vi "Main.vi"(0 "Operations":string(combo), 1 "Delete":bool, 2 "Save":bool, 3 "Load":bool, 5 "Add":bool, 7 "Tree":string(tree), 11 "Error In":errorcluster) -> (15 "Error Out":errorcluster)   [LabVIEW 2023]
doc: "The VI adds the selected the operation into the tree and loads the instances which performs the arithmetic operations and it can save or load the class data into the XML files"
uses:
  Typedef/Queue Operation.ctl
  Typedef/Calculator Data.ctl
  Typedef/Class Data.ctl
  Classes/Arithemtic Operation/Arithemetic Operation.lvclass
  Typedef/DVR Ref.ctl
  Typedef/User Event Operations.ctl
  <vilib>/Utility/xml.llb/Write to XML File(string).vi
  <vilib>/Utility/xml.llb/Read From XML File(array).vi
panel:
  # "Instructions:\n1. Run the VI.\n2. Select the operation to be done from the Operations.\n3. Click Add to create a instance and is added in the tree.\n4. Select the instance name in the tree to load the instance.\n5. Specify the input values in the instance and observe the output\n6. On clicking the Delete button the selected instance will be deleted. \n7. Click Save to save the values all instances in an XML file.\n8. Click Load to load the values of all instances from an XML file.\n9. Click panel close to stop the VI from running."
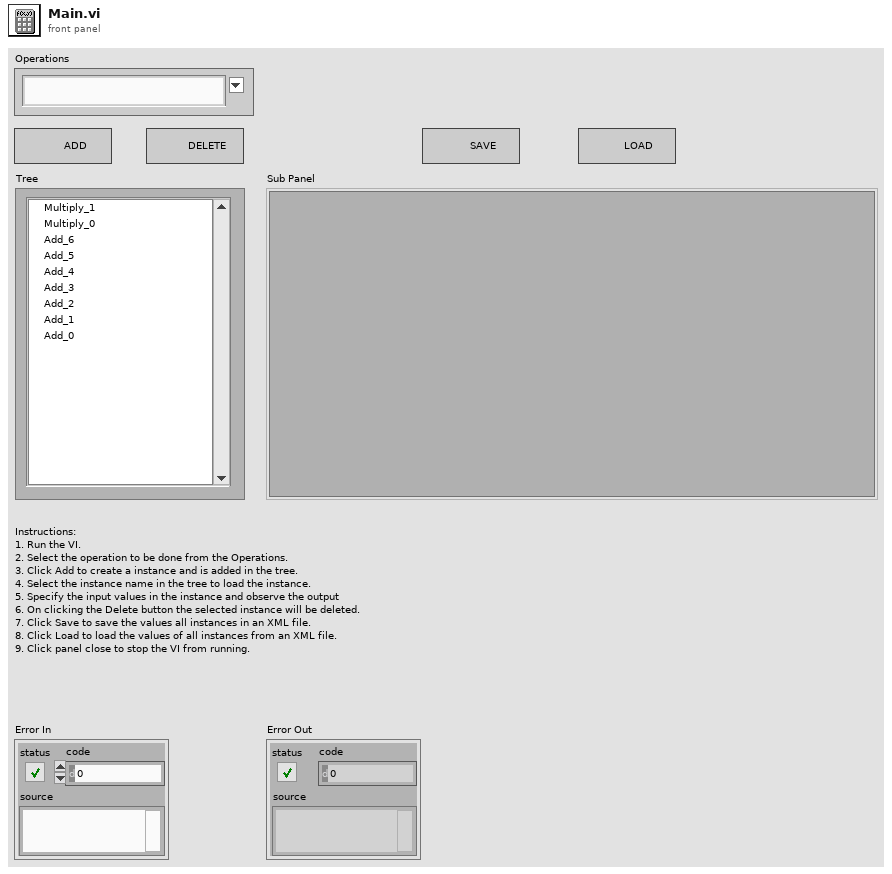
[diagram p1: front panel]
types:
  T1 = typedef "User Event Operations.ctl" = enum16{"Obtain", "Generate", "Release"}
  T2 = typedef "Calculator Data.ctl" = cluster{"Selected Item":string, "Selected Tag":string, "XML Path":path, "Instance Data Array":T3[], "Class Name":string, "Close":refnum<data-value>, "DVR Ref Array":T4[]}
  T3 = typedef "Class Data.ctl" = cluster{"Class Data":refnum<class "Arithemetic Operation.lvclass">, "Name":string}
  T4 = typedef "DVR Ref.ctl" = cluster{"Class Name":string, "DVR":refnum<data-value>}
  T5 = typedef "Queue Operation.ctl" = enum16{"Create & Enqueue N", "Enqueue N", "Dequeue", "Enstack N", "Flush", "Release"}
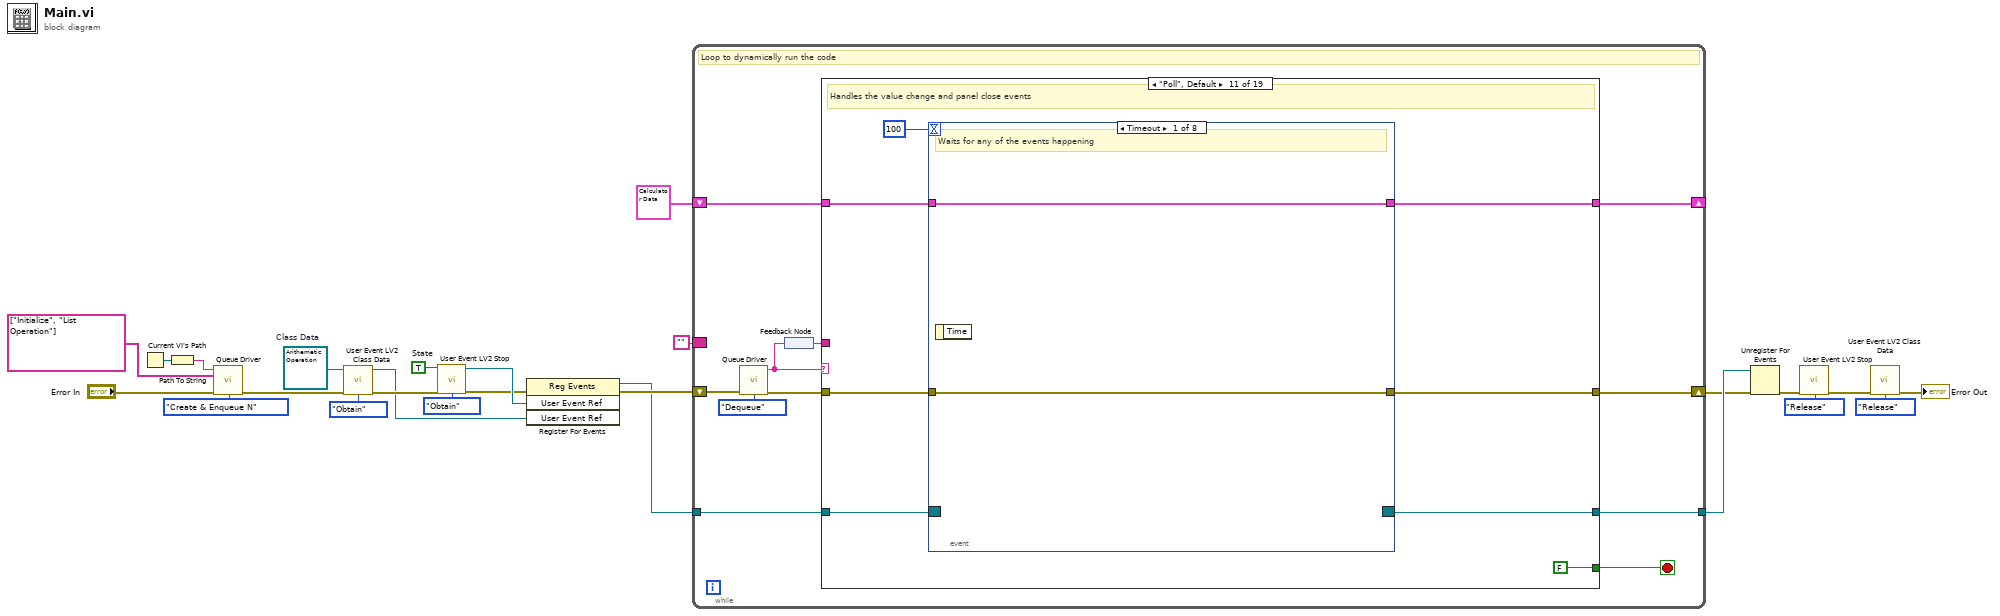
[diagram p0: block diagram]
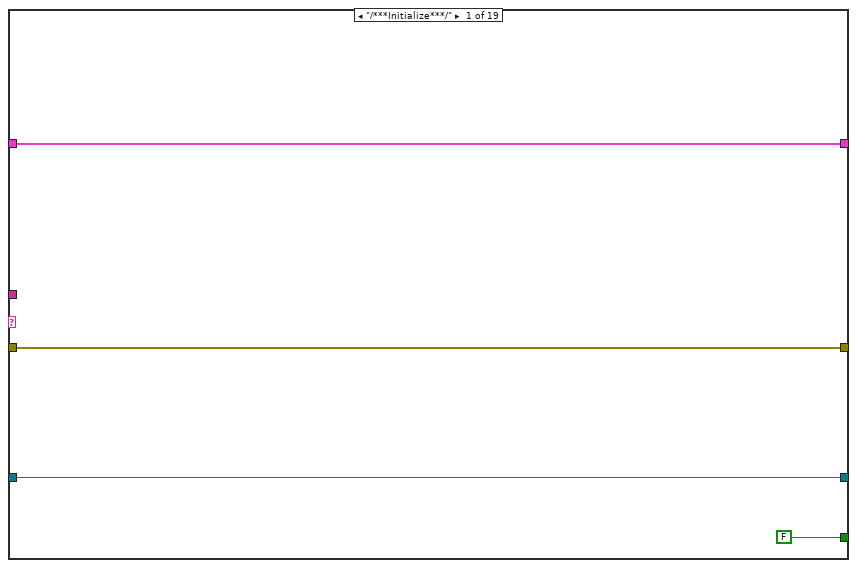
[diagram p2: hidden frame]
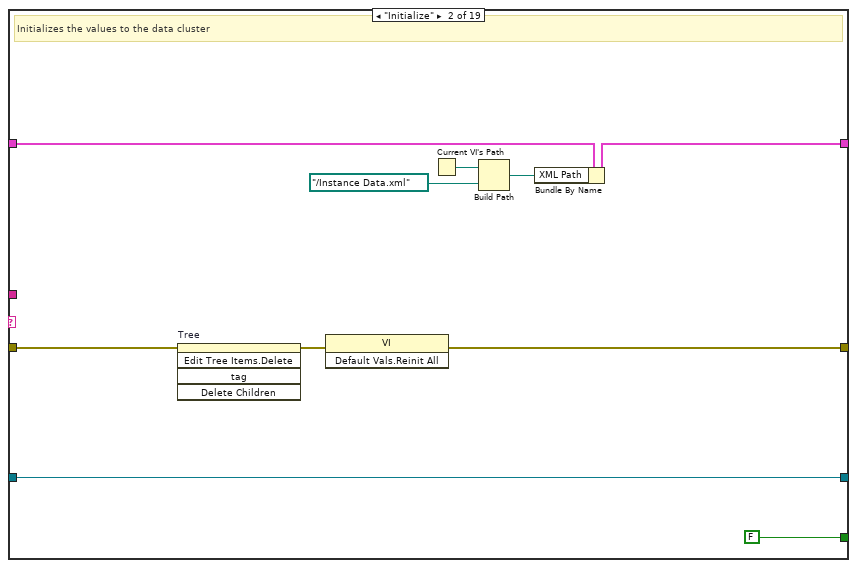
[diagram p3: hidden frame]
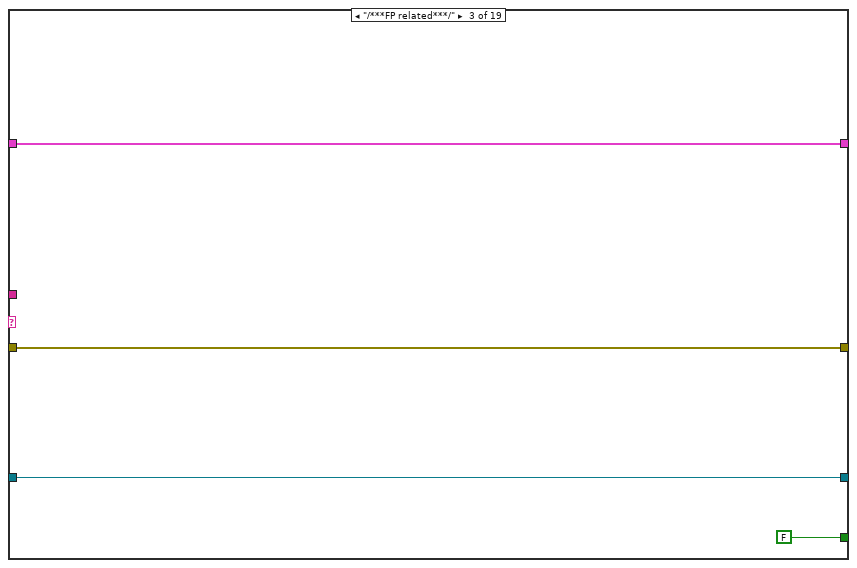
[diagram p4: hidden frame]
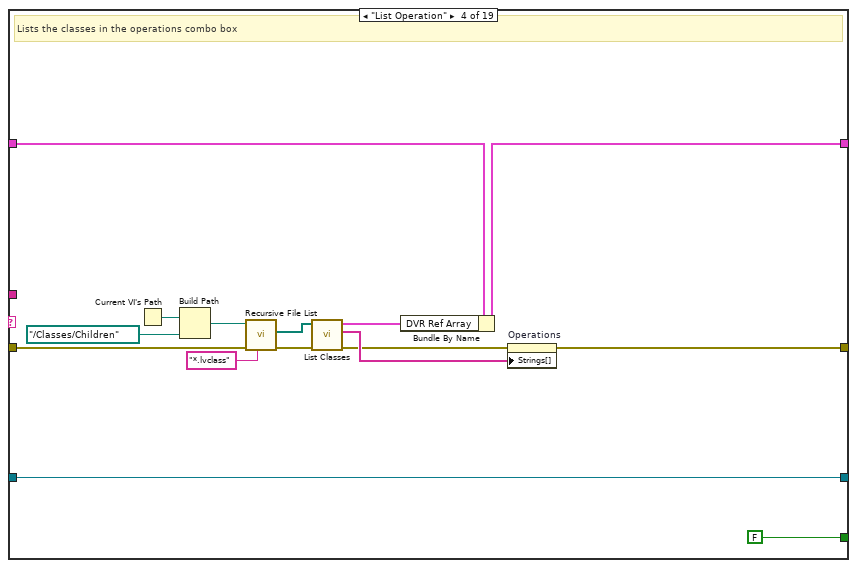
[diagram p5: hidden frame]
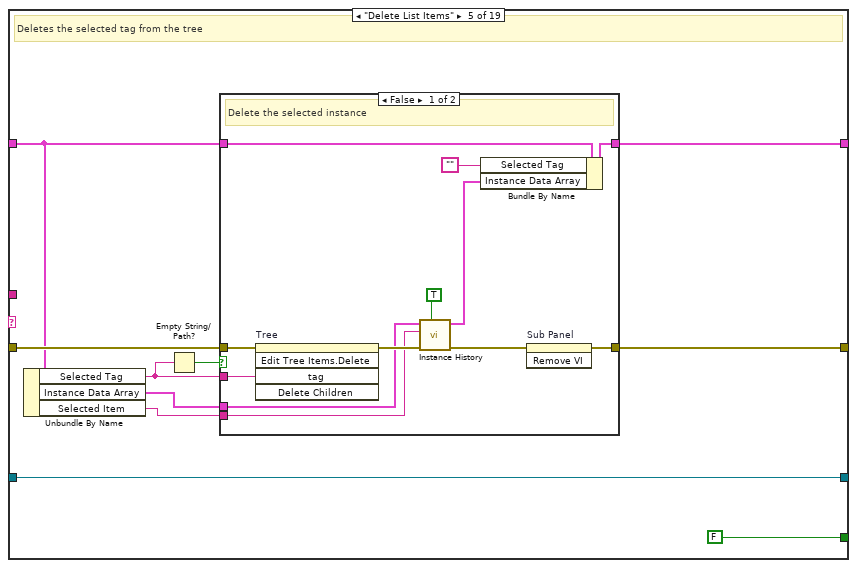
[diagram p6: hidden frame]
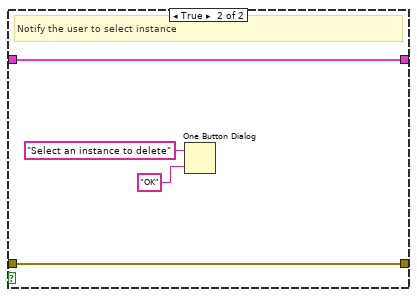
[diagram p7: hidden frame]
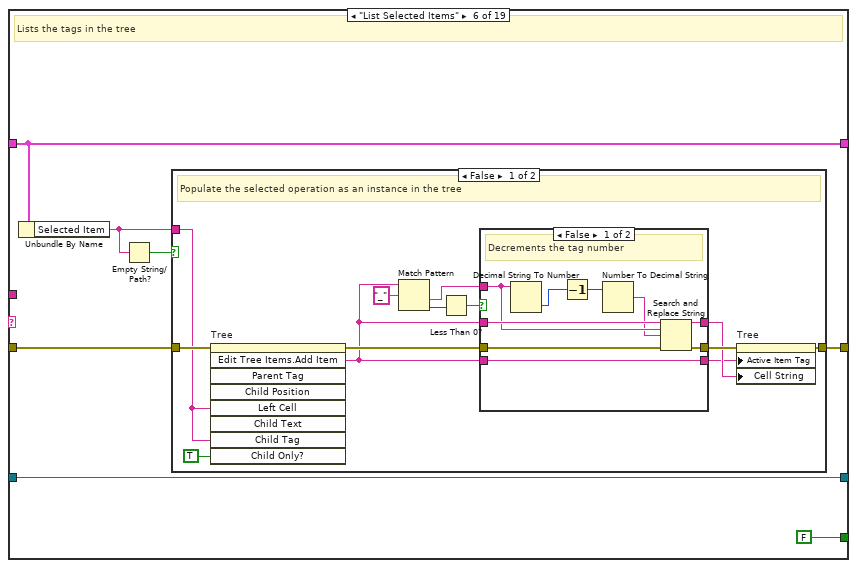
[diagram p8: hidden frame]
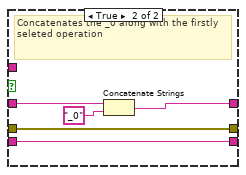
[diagram p9: hidden frame]
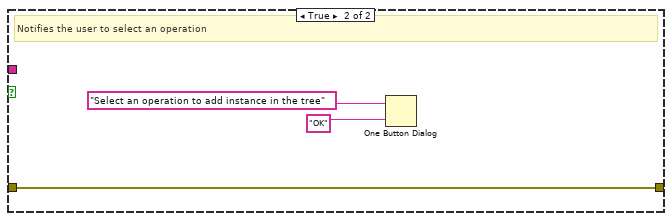
[diagram p10: hidden frame]
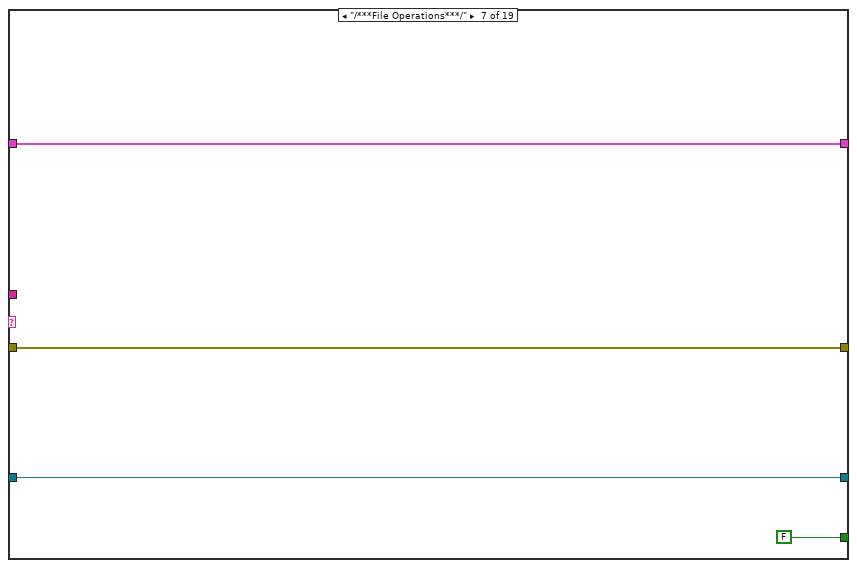
[diagram p11: hidden frame]
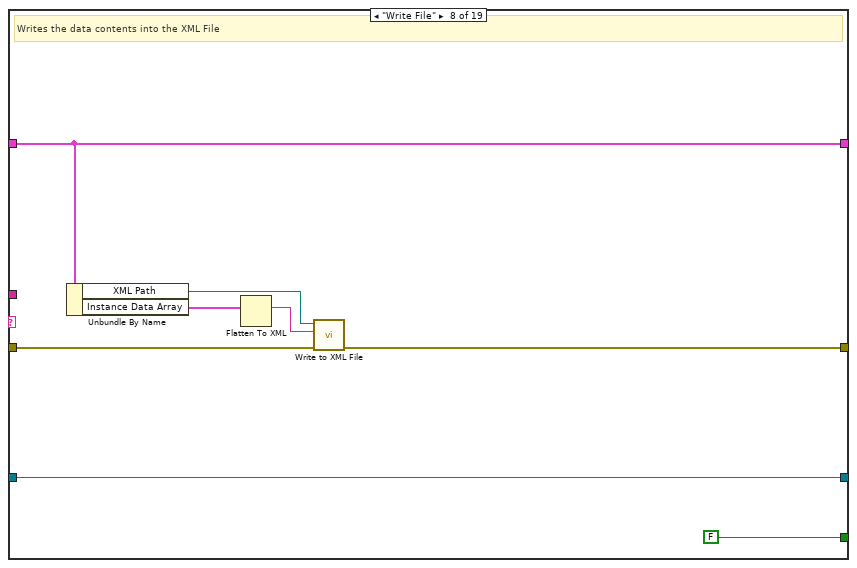
[diagram p12: hidden frame]
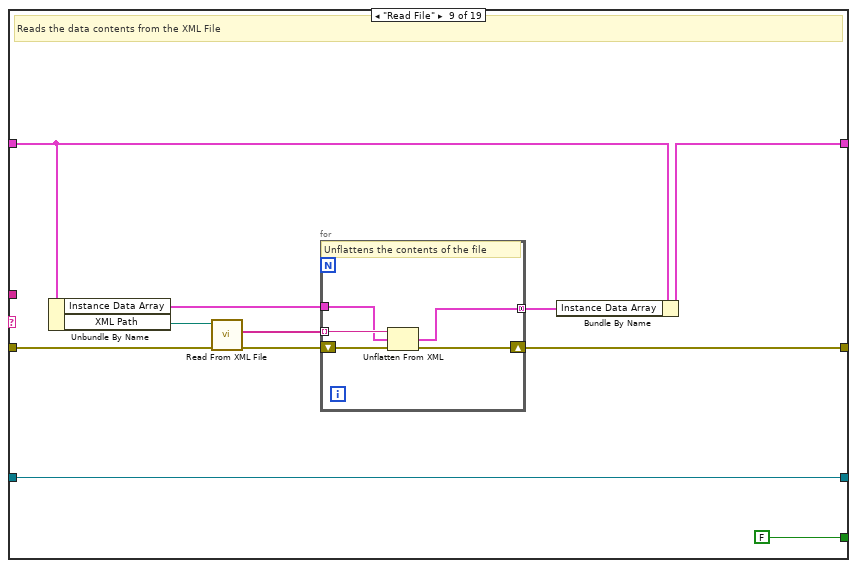
[diagram p13: hidden frame]
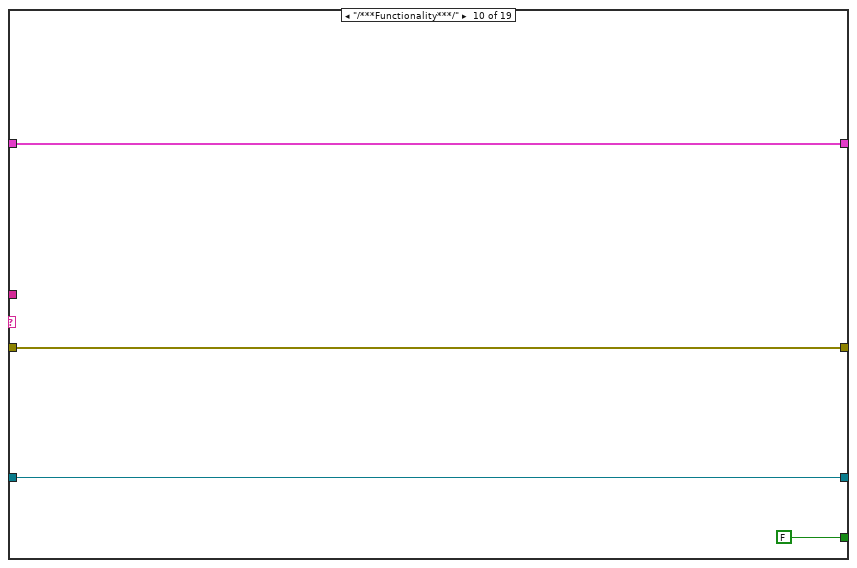
[diagram p14: hidden frame]
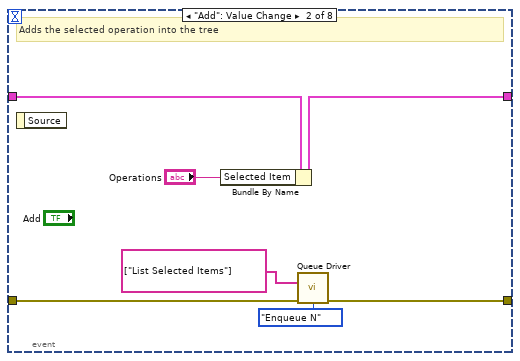
[diagram p15: hidden frame]
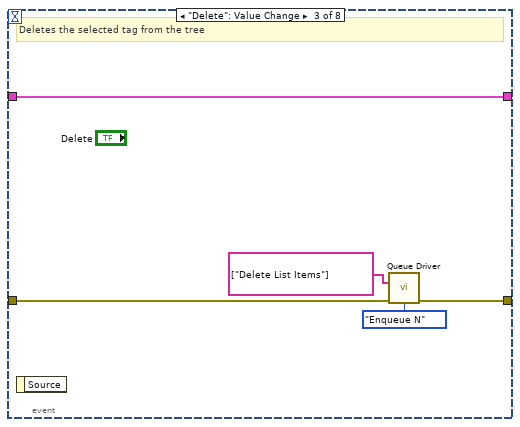
[diagram p16: hidden frame]
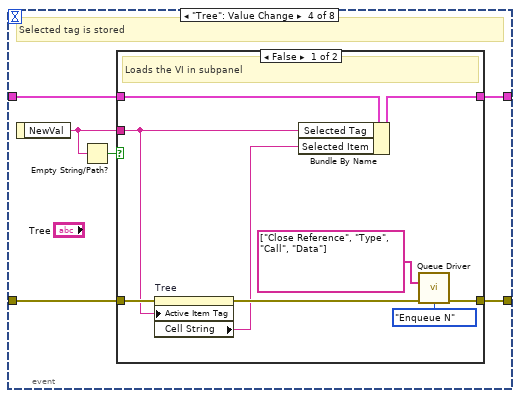
[diagram p17: hidden frame]
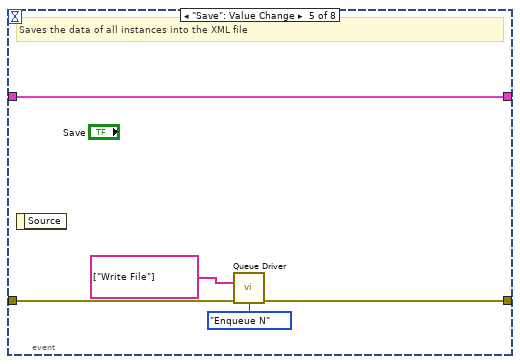
[diagram p19: hidden frame]
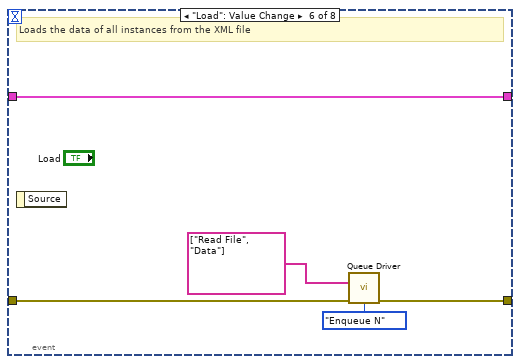
[diagram p20: hidden frame]
diagram:
  w9 = refnum<class "Arithemetic Operation.lvclass"> refnum  # Class Data
  w20 = TRUE  # State
  n1 = Current VI's Path() -> (path=w4:path)
  n2 = Path To String(path=w4) -> (string=w3:string)
  n3 = call "Queue Driver.vi"("Queue Name"=w3, "States[]"=string[] ["Initialize", "List Operation"], "Error In"="Error In", "Queue Operation"=Queue_Operation."Create & Enqueue N") -> ("Error Out"=w23:errorcluster)  [unwired: 10 in, 1 out]
  n4 = call "User Event LV2 Class Data.vi"("Class Data"=w9, "Error In"=w23, "Operation"=User_Event_Operations."Obtain") -> ("User Event Ref"=w17:refnum<user-event>, "Error Out"=w18:errorcluster)  [unwired: 11 in]
  n5 = call "User Event LV2 Stop.vi"("Stop"=w20, "Error In"=w18, "Operation"=User_Event_Operations."Obtain") -> ("User Event Ref"=w8:refnum<user-event>, "Error Out"=w7:errorcluster)  [unwired: 11 in]
  n6 = register-events(error in=w7, w8, w17) -> (reference out=w16:refnum<event-registration>, error out=w19:errorcluster)  [unwired: 1 in]
  n7 = while {
    shift-right: [w32] -> _
    shift-left: T2 {"Selected Item"="", "Selected Tag"="", "XML Path"=path "", "Instance Data Array"=[], "Class Name"="", "Close"=refnum, "DVR Ref Array"=[]} ("Calculator Data") -> [w33]
    border: "" -> [_]
    shift-right: [w34] -> w2
    shift-left: w19 -> [w36]
    tunnel: w16 -> [w27]
    tunnel: [w26] -> w12
    stop <- w31 stop-if-true
    # "Loop to dynamically run the code"
    n8 = call "Queue Driver.vi"("Error In"=w36, "Queue Operation"=Queue_Operation."Dequeue") -> ("Dequeue Element"=w29:string, "Error Out"=w35:errorcluster)  [unwired: 12 in]
    n9 = feedback-in #1(w29) -> ()
    n10 = feedback #1() -> (w30:string)
    n11 = case shown="\"Poll\", Default" w29 {
      tunnel: w35 -> [w40 w50 w54 w66 w79 w102 w136 w144 w155 w164 w172 w239 w248 w259 w266 w282 w289 w308 w311]
      tunnel: [w40 w41 w54 w64 w76 w99 w136 w141 w154 w164 w171 w236 w246 w259 w268 w282 w291 w308 w312] -> w34
      tunnel: w33 -> [w39 w49 w53 w58 w75 w101 w135 w142 w151 w163 w169 w237 w250 w258 w264 w281 w297 w307 w314]
      tunnel: [w39 w45 w53 w57 w74 w101 w135 w142 w147 w163 w168 w237 w250 w257 w270 w281 w297 w307 w314] -> w32
      tunnel: [FALSE ("Stop") FALSE ("Stop") FALSE ("Stop") FALSE ("Stop") FALSE ("Stop") FALSE ("Stop") FALSE ("Stop") FALSE ("Stop") FALSE ("Stop") FALSE ("Stop") FALSE ("Stop") FALSE ("Stop") FALSE ("Stop") FALSE ("Stop") FALSE ("Stop") FALSE ("Stop") FALSE ("Stop") FALSE ("Stop") TRUE ("Stop")] -> w31
      tunnel: w30 -> [_ _ _ _ _ _ _ _ _ _ _ _ _ _ _ _ w285 _ _]
      tunnel: w27 -> [w38 w46 w52 w69 w77 w98 w134 w138 w145 w162 w166 w238 w245 w256 w272 w280 w283 w306 w309]
      tunnel: [w38 w46 w52 w69 w77 w98 w134 w138 w145 w162 w165 w238 w245 w256 w272 w280 w283 w306 w309] -> w26
      frame "/***Initialize***/" {
      }
      frame "Initialize" {
        # "Initializes the values to the data cluster"
        n12 = invoke on="Tree" class="Tree (strict)" method="Edit Tree Items.Delete"(error in=w50) -> (error out=w47:errorcluster)  [unwired: 4 in, 4 out]
        n13 = invoke class="VI" method="Default Vals.Reinit All"(error in=w47) -> (error out=w41:errorcluster)  [unwired: 2 in, 2 out]
        n14 = Current VI's Path() -> (path=w44:path)
        n15 = Build Path(base path=w44, name or relative path=path "../Instance Data.xml") -> (appended path=w42:path)
        n16 = Bundle By Name(cluster=w49, "XML Path"=w42) -> (w45:T2)
      }
      frame "/***FP related***/" {
      }
      frame "List Operation" {
        # "Lists the classes in the operations combo box"
        n17 = Current VI's Path() -> (path=w68:path)
        n18 = Build Path(base path=w68, name or relative path=path "../Classes/Children") -> (appended path=w65:path)
        n19 = call <vilib>:"Recursive File List.vi"("pattern"="*.lvclass", "error in (no error)"=w66, "Folder Path"=w65) -> ("error out"=w60:errorcluster, "All Files in Dir"=w55:path[])  [unwired: 4 in, 3 out]
        n20 = call "List Classes.vi"("Error In"=w60, "Class Path"=w55) -> ("Error Out"=w59:errorcluster, "Class Names"=w63:string[], "DVR Ref"=w56:T4[])  [unwired: 7 in]
        n21 = Bundle By Name(cluster=w58, "DVR Ref Array"=w56) -> (w57:T2)
        n22 = property on="Operations" class="CmbBox"(error in=w59, "Strings[]"=w63) -> (error out=w64:errorcluster)  [unwired: 1 in, 1 out]
      }
      frame "Delete List Items" {
        # "Deletes the selected tag from the tree"
        n23 = Unbundle By Name(w75) -> ("Selected Tag"=w73:string, "Instance Data Array"=w71:T3[], "Selected Item"=w70:string)
        n24 = Empty String/Path?(string/path=w73) -> (empty?=w72:bool)
        n25 = case shown="False" w72 {
          tunnel: w79 -> [w91 w94]
          tunnel: w73 -> [w89 _]
          tunnel: [w88 w94] -> w76
          tunnel: w75 -> [w87 w95]
          tunnel: [w86 w95] -> w74
          tunnel: w71 -> [w83 _]
          tunnel: w70 -> [w82 _]
          frame False {
            # "Delete the selected instance"
            n26 = invoke on="Tree" class="Tree (strict)" method="Edit Tree Items.Delete"(error in=w91, "tag"=w89) -> (error out=w90:errorcluster)  [unwired: 3 in, 4 out]
            n27 = call "Instance History.vi"("Instance Data Array in"=w83, "Selected Instance"=w82, "Error In"=w90, "Delete?"=TRUE) -> ("Instance Data Array out"=w80:T3[], "Error Out"=w84:errorcluster)  [unwired: 5 in]
            n28 = Bundle By Name(cluster=w87, "Selected Tag"="", "Instance Data Array"=w80) -> (w86:T2)
            n29 = invoke on="Sub Panel" class="SubPnl" method="Remove VI"(error in=w84) -> (error out=w88:errorcluster)  [unwired: 2 in, 2 out]
          }
          frame True {
            # "Notify the user to select instance"
            n30 = One Button Dialog(message="Select an instance to delete", button name ("OK")="OK") -> ()  [unwired: 1 out]
          }
        }
      }
      frame "List Selected Items" {
        # "Lists the tags in the tree"
        n31 = Unbundle By Name(w101) -> ("Selected Item"=w96:string)
        n32 = Empty String/Path?(string/path=w96) -> (empty?=w97:bool)
        n33 = case shown="False" w97 {
          tunnel: w102 -> [w115 w132]
          tunnel: w96 -> [w103 _]
          tunnel: [w108 w132] -> w99
          frame False {
            # "Populate the selected operation as an instance in the tree"
            n34 = invoke on="Tree" class="Tree (strict)" method="Edit Tree Items.Add Item"(error in=w115, "Left Cell"=w103, "Child Tag"=w103, "Child Only?"=TRUE) -> (error out=w113:errorcluster, "Edit Tree Items:Add Item"=w106:string)  [unwired: 5 in, 7 out]
            n35 = Match Pattern(string=w106, regular expression="_") -> (after substring=w109:string, offset past match=w112:i32)  [unwired: 1 in, 2 out]
            n36 = Less Than 0?(x=w112) -> (x < 0?=w110:bool)
            n37 = case shown="False" w110 {
              tunnel: w113 -> [w124 w129]
              tunnel: [w123 w129] -> w111
              tunnel: w106 -> [w122 w128]
              tunnel: w109 -> [w121 _]
              tunnel: [w118 w126] -> w107
              tunnel: w106 -> [w116 w125]
              tunnel: [w116 w125] -> w105
              frame False {
                # "Decrements the tag number"
                n38 = Decimal String To Number(string=w121) -> (number=w117:i32)  [unwired: 2 in, 1 out]
                n39 = Decrement(x=w117) -> (x-1=w120:i32)
                n40 = Number To Decimal String(number=w120) -> (decimal integer string=w119:string)  [unwired: 1 in]
                n41 = Search and Replace String(input string=w122, search string=w121, replace string=w119, error in=w124) -> (result string=w118:string, error out=w123:errorcluster)  [unwired: 4 in, 2 out]
              }
              frame True {
                # "Concatenates the _0 along with the firstly seleted operation"
                n42 = Concatenate Strings(w128, "_0" ("string")) -> (w126:string)
              }
            }
            n43 = property on="Tree" class="Tree (strict)"(error in=w111, "Active Item Tag"=w105, "Cell String"=w107) -> (error out=w108:errorcluster)  [unwired: 1 in, 1 out]
          }
          frame True {
            # "Notifies the user to select an operation"
            n44 = One Button Dialog(message="Select an operation to add instance in the tree", button name ("OK")="OK") -> ()  [unwired: 1 out]
          }
        }
      }
      frame "/***File Operations***/" {
      }
      frame "Write File" {
        # "Writes the data contents into the XML File"
        n45 = Unbundle By Name(w142) -> ("XML Path"=w137:path, "Instance Data Array"=w140:T3[])
        n46 = Flatten To XML(6:w140) -> (2:w139:string)
        n47 = call-poly <vilib>:"Write to XML File.vi"("error in (no error)"=w144, "XML Input"=w139, "XML File Path"=w137) -> ("error out"=w141:errorcluster)  [unwired: 6 in, 2 out]
      }
      frame "Read File" {
        # "Reads the data contents from the XML File"
        n48 = Unbundle By Name(w151) -> ("Instance Data Array"=w148:T3[], "XML Path"=w150:path)
        n49 = call-poly <vilib>:"Read From XML File.vi"("error in (no error)"=w155, "XML File Path"=w150) -> ("error out"=w152:errorcluster, "XML Elements"=w149:string[])  [unwired: 7 in, 1 out]
        n50 = for {
          tunnel: w149 -> [w158] mode=indexing
          shift-right: [w160] -> w154
          shift-left: w152 -> [w159]
          tunnel: w148 -> [w157]
          tunnel: [w156] -> w146 mode=concatenating
          # "Unflattens the contents of the file"
          n51 = Unflatten From XML(xml string=w158, type=w157, error in (no error)=w159) -> (value=w156:T3[], error out=w160:errorcluster)
        }
        n52 = Bundle By Name(cluster=w151, "Instance Data Array"=w146) -> (w147:T2)
      }
      frame "/***Functionality***/" {
      }
      frame "Poll", Default {
        # "Handles the value change and panel close events"
        n53 = event shown="[0] Timeout" {
          selector: w166 -> [_ _ _ _ _ _ _ _]
          dyn-events: [_ _ _ _ _ _ _ _] -> w165
          timeout: 100 -> [_ _ _ _ _ _ _ _]
          tunnel: w172 -> [w174 w179 w186 w192 w206 w211 w216 w226]
          tunnel: [w174 w178 w185 w189 w205 w210 w221 w225] -> w171
          tunnel: w169 -> [w173 w181 w184 w191 w208 w213 w215 w232]
          tunnel: [w173 w177 w184 w190 w208 w213 w215 w228] -> w168
          event Timeout {
            # "Waits for any of the events happening"
            n54 = event-data() -> ()  [unwired: 1 in, 1 out]
          }
          event "Add": Value Change {
            # "Adds the selected operation into the tree"
            n55 = event-data() -> ()  [unwired: 1 in, 1 out]
            n56 = Bundle By Name(cluster=w181, "Selected Item"="Operations") -> (w177:T2)
            n57 = call "Queue Driver.vi"("States[]"=string[] ["List Selected Items"] ("Array of States"), "Error In"=w179, "Queue Operation"=Queue_Operation."Enqueue N") -> ("Error Out"=w178:errorcluster)  [unwired: 11 in, 1 out]
          }
          event "Delete": Value Change {
            # "Deletes the selected tag from the tree"
            n58 = event-data() -> ()  [unwired: 1 in, 1 out]
            n59 = call "Queue Driver.vi"("States[]"=string[] ["Delete List Items"] ("Array of States"), "Error In"=w186, "Queue Operation"=Queue_Operation."Enqueue N") -> ("Error Out"=w185:errorcluster)  [unwired: 11 in, 1 out]
          }
          event "Tree": Value Change {
            # "Selected tag is stored"
            n60 = event-data() -> ("NewVal"=w187:string)  [unwired: 1 in]
            n61 = Empty String/Path?(string/path=w187) -> (empty?=w188:bool)
            n62 = case shown="False" w188 {
              tunnel: w192 -> [w201 w202]
              tunnel: w191 -> [w200 w203]
              tunnel: [w199 w203] -> w190
              tunnel: [w198 w202] -> w189
              tunnel: w187 -> [w193 _]
              frame False {
                # "Loads the VI in subpanel"
                n63 = property on="Tree" class="Tree (strict)"(error in=w201, "Active Item Tag"=w193) -> (error out=w195:errorcluster, "Cell String"=w194:string)  [unwired: 1 in, 1 out]
                n64 = Bundle By Name(cluster=w200, "Selected Tag"=w193, "Selected Item"=w194) -> (w199:T2)
                n65 = call "Queue Driver.vi"("States[]"=string[] ["Close Reference", "Type", "Call", "Data"] ("Array of States"), "Error In"=w195, "Queue Operation"=Queue_Operation."Enqueue N") -> ("Error Out"=w198:errorcluster)  [unwired: 11 in, 1 out]
              }
              frame True {
              }
            }
          }
          event "Save": Value Change {
            # "Saves the data of all instances into the XML file"
            n66 = event-data() -> ()  [unwired: 1 in, 1 out]
            n67 = call "Queue Driver.vi"("States[]"=string[] ["Write File"] ("Array of States"), "Error In"=w206, "Queue Operation"=Queue_Operation."Enqueue N") -> ("Error Out"=w205:errorcluster)  [unwired: 11 in, 1 out]
          }
          event "Load": Value Change {
            # "Loads the data of all instances from the XML file"
            n68 = event-data() -> ()  [unwired: 1 in, 1 out]
            n69 = call "Queue Driver.vi"("States[]"=string[] ["Read File", "Data"] ("Array of States"), "Error In"=w211, "Queue Operation"=Queue_Operation."Enqueue N") -> ("Error Out"=w210:errorcluster)  [unwired: 11 in, 1 out]
          }
          event Panel Close? {
            w220 = TRUE  # State
            # "Enqueues the exit state to stop the VI running"
            n70 = event-data() -> ()  [unwired: 1 in, 1 out]
            n71 = Unbundle By Name(w215) -> ("DVR Ref Array"=w217:T4[])
            n72 = call "Delete DVR.vi"("Error In"=w216, "DVR Ref Array"=w217) -> ("Error out"=w214:errorcluster)  [unwired: 9 in]
            n73 = call "Queue Driver.vi"("States[]"=string[] ["Exit"] ("Array of States"), "Error In"=w214, "Queue Operation"=Queue_Operation."Enqueue N") -> ("Error Out"=w223:errorcluster)  [unwired: 11 in, 1 out]
            n74 = call "User Event LV2 Stop.vi"("Stop"=w220, "Error In"=w223, "Operation"=User_Event_Operations."Generate") -> ("Error Out"=w221:errorcluster)  [unwired: 11 in, 1 out]
            n75 = event-data("Discard?"=TRUE) -> ()  [unwired: 1 in, 1 out]
          }
          event User Event {
            # "Stores the instance data"
            n76 = event-data() -> ("Arithemetic Operation.lvclass"=w231:refnum<class "Arithemetic Operation.lvclass">)  [unwired: 1 in]
            n77 = Unbundle By Name(w232) -> ("Instance Data Array"=w230:T3[], "Selected Item"=w229:string)
            n78 = call "Instance History.vi"("Instance Data Array in"=w230, "Selected Instance"=w229, "Class Data"=w231, "Error In"=w226) -> ("Instance Data Array out"=w227:T3[], "Error Out"=w225:errorcluster)  [unwired: 5 in]
            n79 = Bundle By Name(cluster=w232, "Instance Data Array"=w227) -> (w228:T2)
          }
        }
      }
      frame "Close Reference" {
        # "Closes the asynchronous call reference of the previous instance"
        n80 = Unbundle By Name(w237) -> ("Close"=w233:refnum<data-value>)
        n81 = Not A Number/Path/Refnum?(number/path/refnum=w233) -> (NaN/Path/Refnum?=w234:bool)
        n82 = case shown="False" w234 {
          tunnel: w239 -> [w242 w243]
          tunnel: [w241 w243] -> w236
          tunnel: w233 -> [w240 _]
          frame False {
            # "Close the VI reference"
            n83 = call "Close Ref.vi"("Error In"=w242, "DVR Ref"=w240) -> ("Error Out"=w241:errorcluster)  [unwired: 9 in]
          }
          frame True {
          }
        }
      }
      frame "Data" {
        # "Loads the class data for the selected instance"
        n84 = Unbundle By Name(w250) -> ("Instance Data Array"=w249:T3[], "Selected Item"=w244:string)
        n85 = call "get Class Data.vi"("Error In"=w248, "Selected Instance"=w244, "Instance Data Array"=w249) -> ("Error Out"=w246:errorcluster)  [unwired: 8 in]
      }
      frame "Type" {
        # "Updates the class name based on the selected tag"
        n86 = Unbundle By Name(w258) -> ("Selected Tag"=w255:string)
        n87 = Match Pattern(string=w255, regular expression="_") -> (before substring=w253:string)  [unwired: 1 in, 3 out]
        n88 = Concatenate Strings(w253, ".lvclass" ("string")) -> (w251:string)
        n89 = Bundle By Name(cluster=w258, "Class Name"=w251) -> (w257:T2)
      }
      frame "Call" {
        # "Calls the selected operation UI"
        n90 = Unbundle By Name(w264) -> ("DVR Ref Array"=w261:T4[], "Class Name"=w263:string)
        n91 = for {
          shift-right: [w278] -> w265
          shift-left: w266 -> [w278]
          tunnel: w261 -> [w274] mode=indexing
          tunnel: w263 -> [w277]
          tunnel: [w276] -> w262 if=w275
          stop <- w275 stop-if-true
          # "Searches the reference for the respective class"
          n92 = Unbundle By Name(w274) -> ("DVR"=w276:refnum<data-value>, "Class Name"=w273:string)
          n93 = Equal?(x=w273, y=w277) -> (x = y?=w275:bool)
        }
        n94 = control-ref of="Sub Panel"() -> (w269:refnum<vi>)
        n95 = call "Caller DVR.vi"("DVR In"=w262, "Sub Panel"=w269, "Error In"=w265) -> ("DVR Out"=w267:refnum<data-value>, "Error Out"=w268:errorcluster)  [unwired: 11 in]
        n96 = Bundle By Name(cluster=w264, "Close"=w267) -> (w270:T2)
      }
      frame "/***Error***/" {
      }
      frame "Error" {
        # "Displays the error encountered and acts according to user acknowledgement"
        n97 = Unbundle By Name(w289) -> ("code"=w288:i32, "source"=w287:string)
        n98 = call <vilib>:"Clear Errors.vi"("error in (no error)"=w289) -> ("error out"=w294:errorcluster)  [unwired: 5 in, 1 out]
        n99 = Format Into String(format string="Error occurred in state \"%s\"!!\nError Code: %d\nError Source: %s\n\nDo you wish to continue?", error in=w294, w285, w288, w287) -> (resulting string=w295:string, error out=w290:errorcluster)  [unwired: 1 in]
        n100 = Two Button Dialog(message=w295, 1:"Exit" ("F button name (\"Cancel\")"), 2:"Continue" ("T button name (\"OK\")")) -> (T button?=w296:bool)
        n101 = case "Continue?" shown="False" w296 {
          tunnel: [w303 w304] -> w291
          tunnel: w290 -> [w300 w304]
          frame False {
            # "Enqueues the exit state to stop the VI running"
            n102 = call "Queue Driver.vi"("Error In"=w300, "Queue Operation"=Queue_Operation."Flush") -> ("Error Out"=w299:errorcluster)  [unwired: 12 in, 1 out]
            n103 = call "Queue Driver.vi"("States[]"=string[] ["Exit"] ("Array of States"), "Error In"=w299, "Queue Operation"=Queue_Operation."Enqueue N") -> ("Error Out"=w303:errorcluster)  [unwired: 11 in, 1 out]
          }
          frame True {
            # "Continues the VI running"
          }
        }
      }
      frame "/***Exit***/" {
      }
      frame "Exit" {
        # "Stops the VI running"
        n104 = call "Queue Driver.vi"("Error In"=w311, "Queue Operation"=Queue_Operation."Release") -> ("Error Out"=w312:errorcluster)  [unwired: 12 in, 1 out]
      }
    }
  }
  n105 = Unregister For Events(event registration refnum=w12, error in=w2) -> (error out=w15:errorcluster)
  n106 = call "User Event LV2 Stop.vi"("Error In"=w15, "Operation"=User_Event_Operations."Release") -> ("Error Out"=w14:errorcluster)  [unwired: 12 in, 1 out]
  n107 = call "User Event LV2 Class Data.vi"("Error In"=w14, "Operation"=User_Event_Operations."Release") -> ("Error Out"=→"Error Out":errorcluster)  [unwired: 12 in, 1 out]
